vi "Get Object from Variant.vi"(8 "error in (no error)":errorcluster, 11 "LabVIEW Class Path":path) -> (0 "error out":errorcluster, 2 "Object":refnum<class>, 3 "Found?":bool)   [LabVIEW 2014, in "SLL Class.lvlib"]
doc: "This method gets the class object from the Variant LUT."
uses:
  SLL Class.lvlib
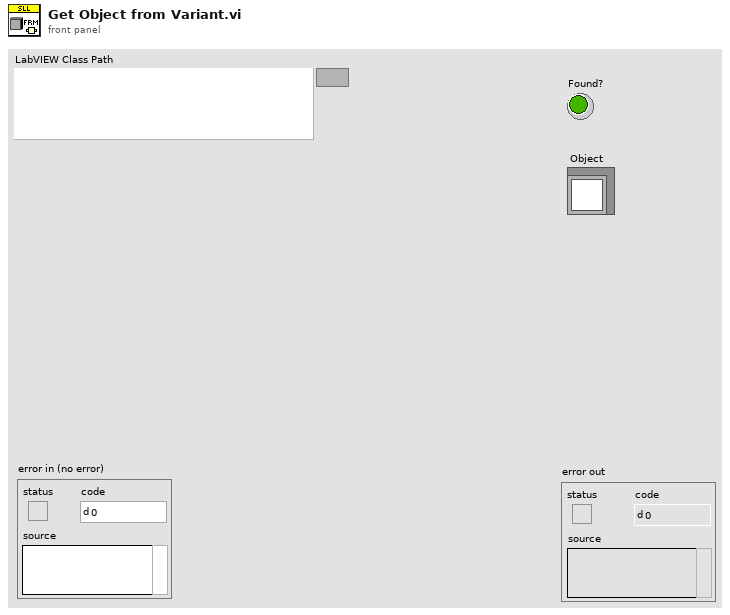
[diagram p1: front panel]
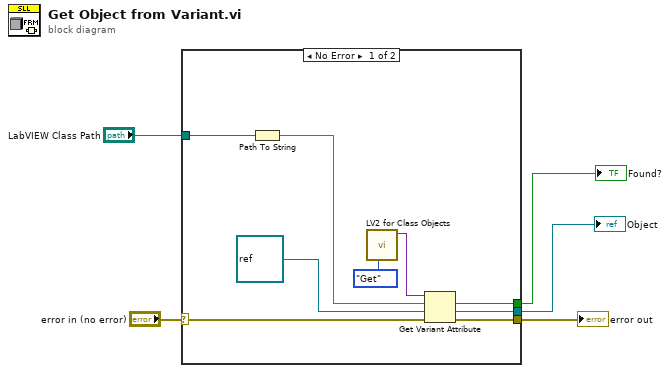
[diagram p0: block diagram]
diagram:
  n1 = case shown="No Error" "error in (no error)" {
    selector: "error in (no error)" -> [w13 w15]
    tunnel: "LabVIEW Class Path" -> [w11 _]
    tunnel: [w8 _] -> w3
    tunnel: [w7 w15] -> w2
    tunnel: [w6 _] -> w1
    frame No Error {
      n2 = Path To String(path=w11) -> (string=w10:string)
      n3 = call "LV2 for Class Objects.vi"("Command"=enum16{"Get", "Set"}."Get") -> ("Variant Out"=w9:variant)  [unwired: 10 in]
      n4 = Get Variant Attribute(Variant=w9, name=w10, default value (empty Variant)=refnum<class> refnum ("Object"), error in=w13) -> (found=w6:bool, value=w8:refnum<class>, error out=w7:errorcluster)  [unwired: 1 out]
    }
    frame Error {
    }
  }
  "Object" <- w3
  "error out" <- w2
  "Found?" <- w1
